vi "Fpga_v6.vi"() -> ()   [LabVIEW 2015]
uses:
  <vilib>/rvi/Emulation/niFpgaGetClockAttributes.vi
  <vilib>/rvi/Emulation/niFpgaSctlEmulationGetInTimedLoop.vi
  <vilib>/rvi/Emulation/niFpgaEmulationReportErrorSimple.vi
  <vilib>/rvi/eio/common/nirviEmuTemplateMethod_errors.vi
  <vilib>/rvi/Emulation/niFpgaCriticalErrorInLSC.vi
  <vilib>/eio/EIONode/EIONode.xnode
panel:
  out "on 2":bool
  out "on":bool
  out "Mod2/DIO6_B":bool
  in  "stop":bool
  in  "Data write ON/OFF":bool
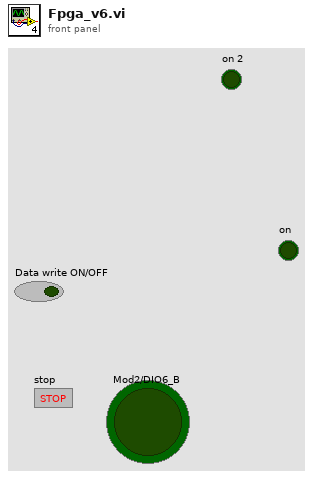
[diagram p1: front panel]
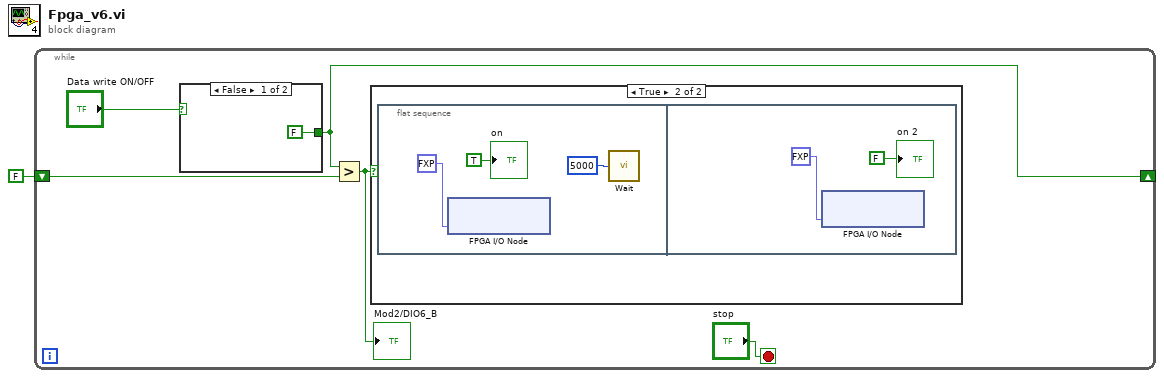
[diagram p0: block diagram]
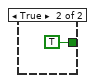
[diagram p3: hidden frame]
diagram:
  n1 = while {
    shift-right: [w5] -> _
    shift-left: FALSE -> [w6]
    stop <- "stop" stop-if-true
    n2 = case shown="False" "Data write ON/OFF" {
      tunnel: [FALSE ("Mod2/DIO6") TRUE ("Mod2/DIO6")] -> w5
      frame False {
      }
      frame True {
      }
    }
    n3 = Greater?(x=w5, y=w6) -> (0:w2:bool)
    "Mod2/DIO6_B" <- w2
    n4 = case shown="True" w2 {
      frame False {
      }
      frame True {
        n5 = flat-sequence {
          frame #0 {
            n6 = xnode "FPGA I/O Node"("Mod4/AO0"=fxp<+/-,20,5> 8.0) -> ()  [unwired: 1 in, 1 out]
            n7 = call "Wait"("Count(mSec)"=u32 5000) -> ()  [unwired: 1 out]
            "on" <- TRUE ("on")
          }
          frame #1 {
            n8 = xnode "FPGA I/O Node"("Mod4/AO0"=fxp<+/-,20,5> 0.0) -> ()  [unwired: 1 in, 1 out]
            "on 2" <- FALSE ("off")
          }
        }
      }
    }
  }
